vi "lzx.vi"() -> ()   [LabVIEW 2017]
uses:
  <vilib>/express/express arith-compare/Formula/XNode/ExpressFormulaBlockNode.xnode
panel:
  in  "数组":void[](array[numeric])
  in  "枚举":enum16{""}(ring)
  in  "下拉列表":u16(ring) items=["合肥", "北京", "重庆", "上海", ""]
  out "转换成年份":dbl[unit]
  in  "带单位的数值":dbl[unit]
  out "数值 2":dbl
  out "数值表示法":dbl format="%<%Y-%m-%d %H:%M:%S>T"
  # "="
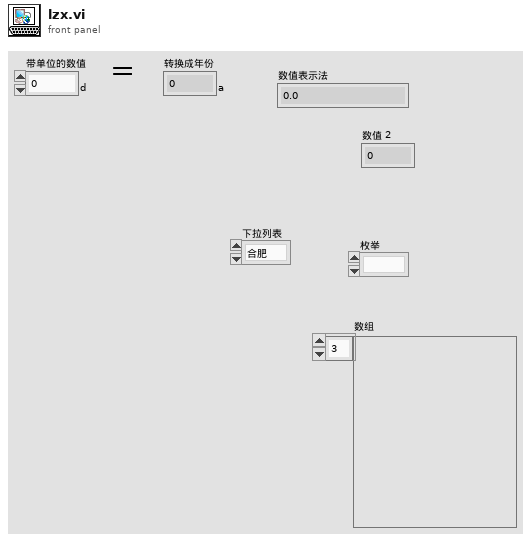
[diagram p1: front panel]
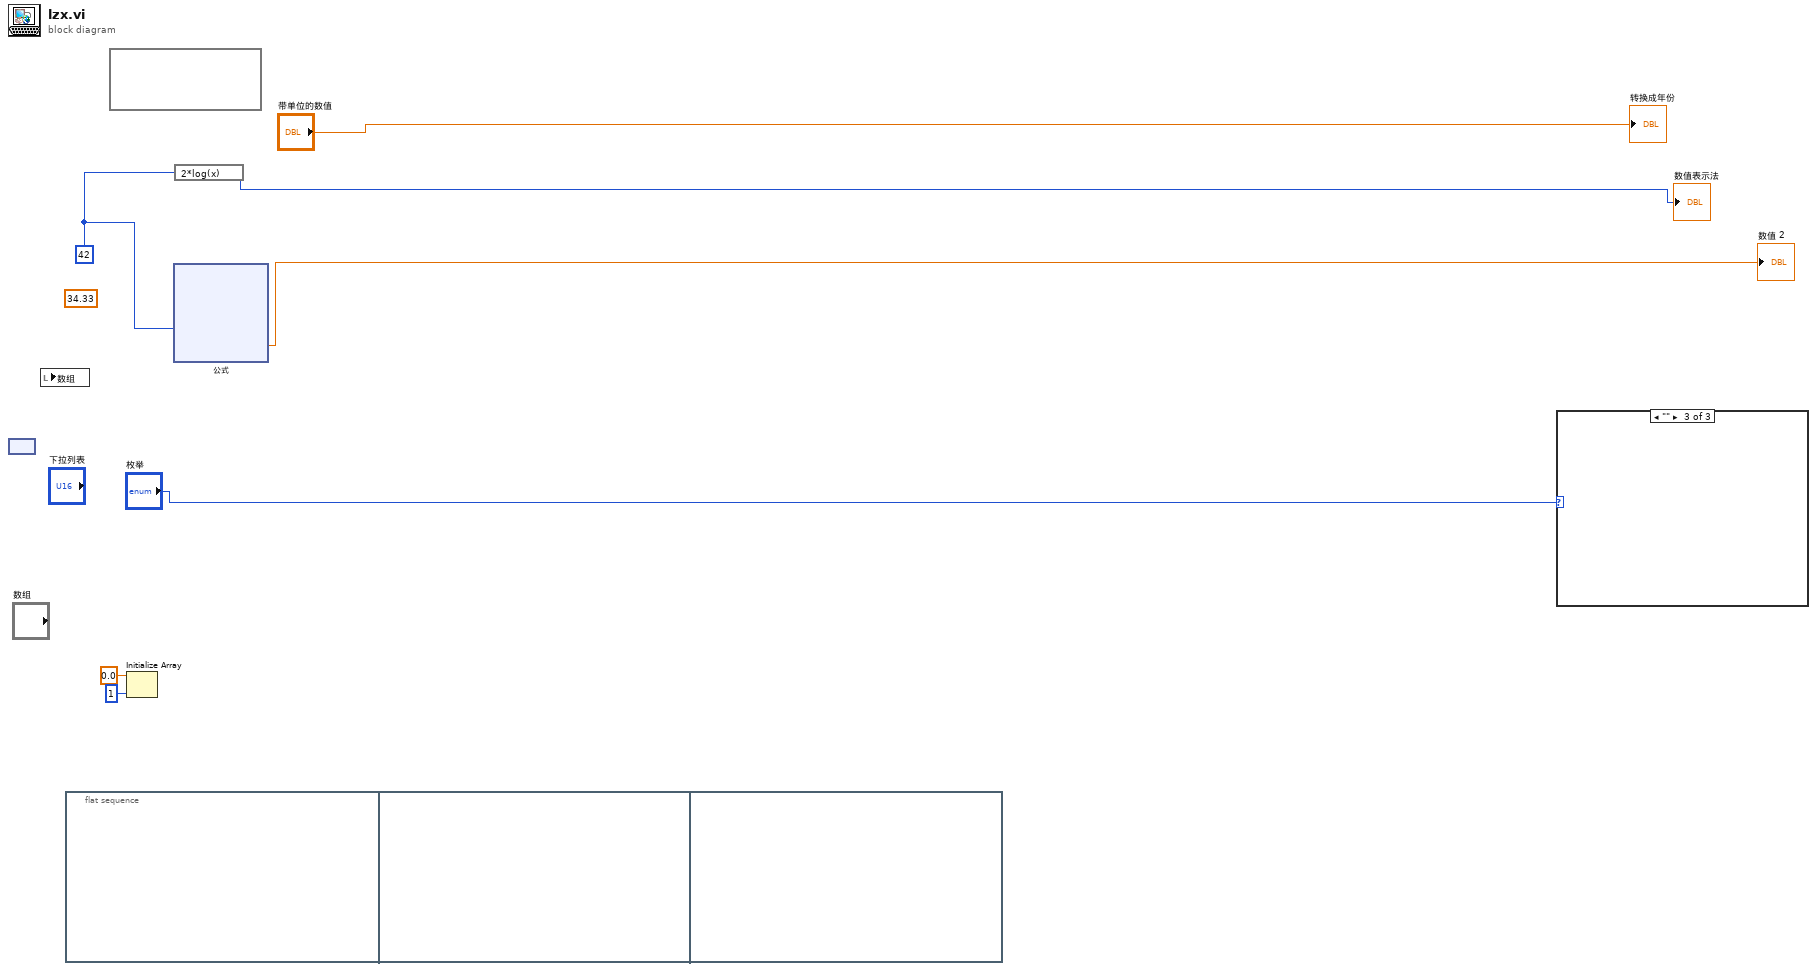
[diagram p0: block diagram]
diagram:
  (unwired) 34.33
  w6 = 42
  n1 = node() -> ()  [unwired: 1 in, 1 out]
  n2 = local read "数组"() -> ()  [unwired: 1 in]
  n3 = flat-sequence {
    frame #0 {
    }
    frame #1 {
    }
    frame #2 {
    }
  }
  n4 = formula code=""() -> ()
  n5 = Initialize Array(0.0 ("元素"), 1 ("维数大小")) -> ()  [unwired: 1 out]
  n6 = xnode "公式"("X1"=w6) -> ("结果"=→"数值 2":dbl)  [unwired: 1 in, 1 out]
  n7 = expression code="2*log(x)"(w6) -> (→"数值表示法":i32)
  n8 = case shown="\"\"" "枚举" {
    frame "", Default {
    }
    frame 1 {
    }
    frame "" {
    }
  }
  "转换成年份" <- "带单位的数值"
